vi "Get Date Time.vi"(8 "error in":errorcluster) -> (0 "error out":errorcluster, 3 "date time":string)   [LabVIEW 2014, in "lvprj2html.lvlib"]
uses:
  lvprj2html.lvlib
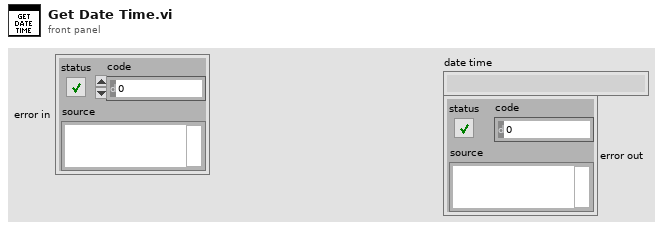
[diagram p1: front panel]
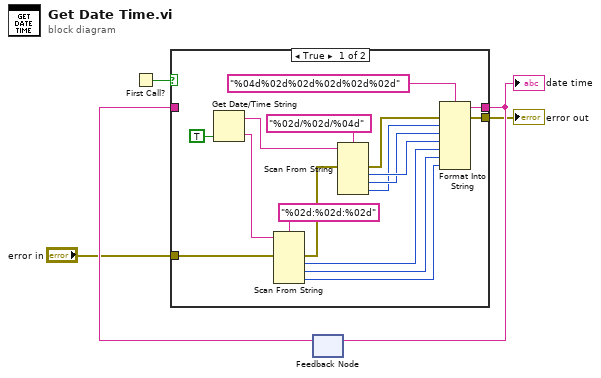
[diagram p0: block diagram]
diagram:
  n1 = First Call?() -> (First Call?: T/F=w3:bool)
  n2 = feedback #1() -> (w4:string)  [unwired: 1 in]
  n3 = case shown="True" w3 {
    tunnel: [w20 w24] -> w5
    tunnel: w4 -> [_ w24]
    tunnel: "error in" -> [w9 w23]
    tunnel: [w6 w23] -> w1
    frame True {
      n4 = Get Date/Time String(want seconds? (F)=TRUE) -> (date string=w18:string, time string=w13:string)  [unwired: 2 in]
      n5 = Scan From String(format string="%02d:%02d:%02d", input string=w13, error in=w9) -> (error out=w8:errorcluster, output 1=w12:i32, output 2=w11:i32, output 3=w10:i32)  [unwired: 4 in, 2 out]
      n6 = Scan From String(format string="%02d/%02d/%04d", input string=w18, error in=w8) -> (error out=w7:errorcluster, output 1=w17:i32, output 2=w16:i32, output 3=w15:i32)  [unwired: 4 in, 2 out]
      n7 = Format Into String(format string="%04d%02d%02d%02d%02d%02d" ("initial string"), error in=w7, w15, w16, w17, w12, w11, w10) -> (resulting string=w20:string, error out=w6:errorcluster)  [unwired: 1 in]
    }
    frame False {
    }
  }
  "date time" <- w5
  "error out" <- w1
  n8 = feedback-in #1(w5) -> ()
